vi "Compute DistanceToTarget2.vi"(8 "Rect":T1, 9 "Camera Type":T3, 11 "Image Src":T2) -> (2 "Distance (ft)":dbl, 3 "Image Dst Out":T2)   [LabVIEW 2025]
doc: "Using the camera lens information and the real world size of the target, use trig and ratios to determine the distance to the target. Also returns the location relative to the image center in a (-1 , 1) coordinate system that may be useful for steering the robot."
uses:
  Camera Types.ctl
  <vilib>/vision/Image Controls.llb/IMAQ Image.ctl
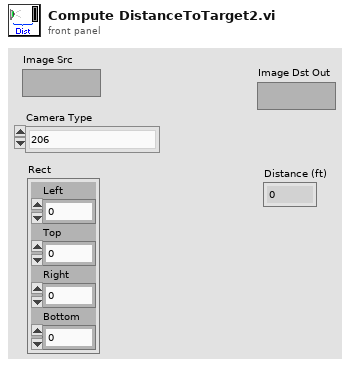
[diagram p1: front panel]
types:
  T1 = cluster{"Left":dbl, "Top":dbl, "Right":dbl, "Bottom":dbl}
  T2 = typedef "IMAQ Image.ctl" = refnum<image>
  T3 = typedef "Camera Types.ctl" = enum16{"206", "1011", "1013", "MS HD3000 square", "MS HD3000 640x480"}
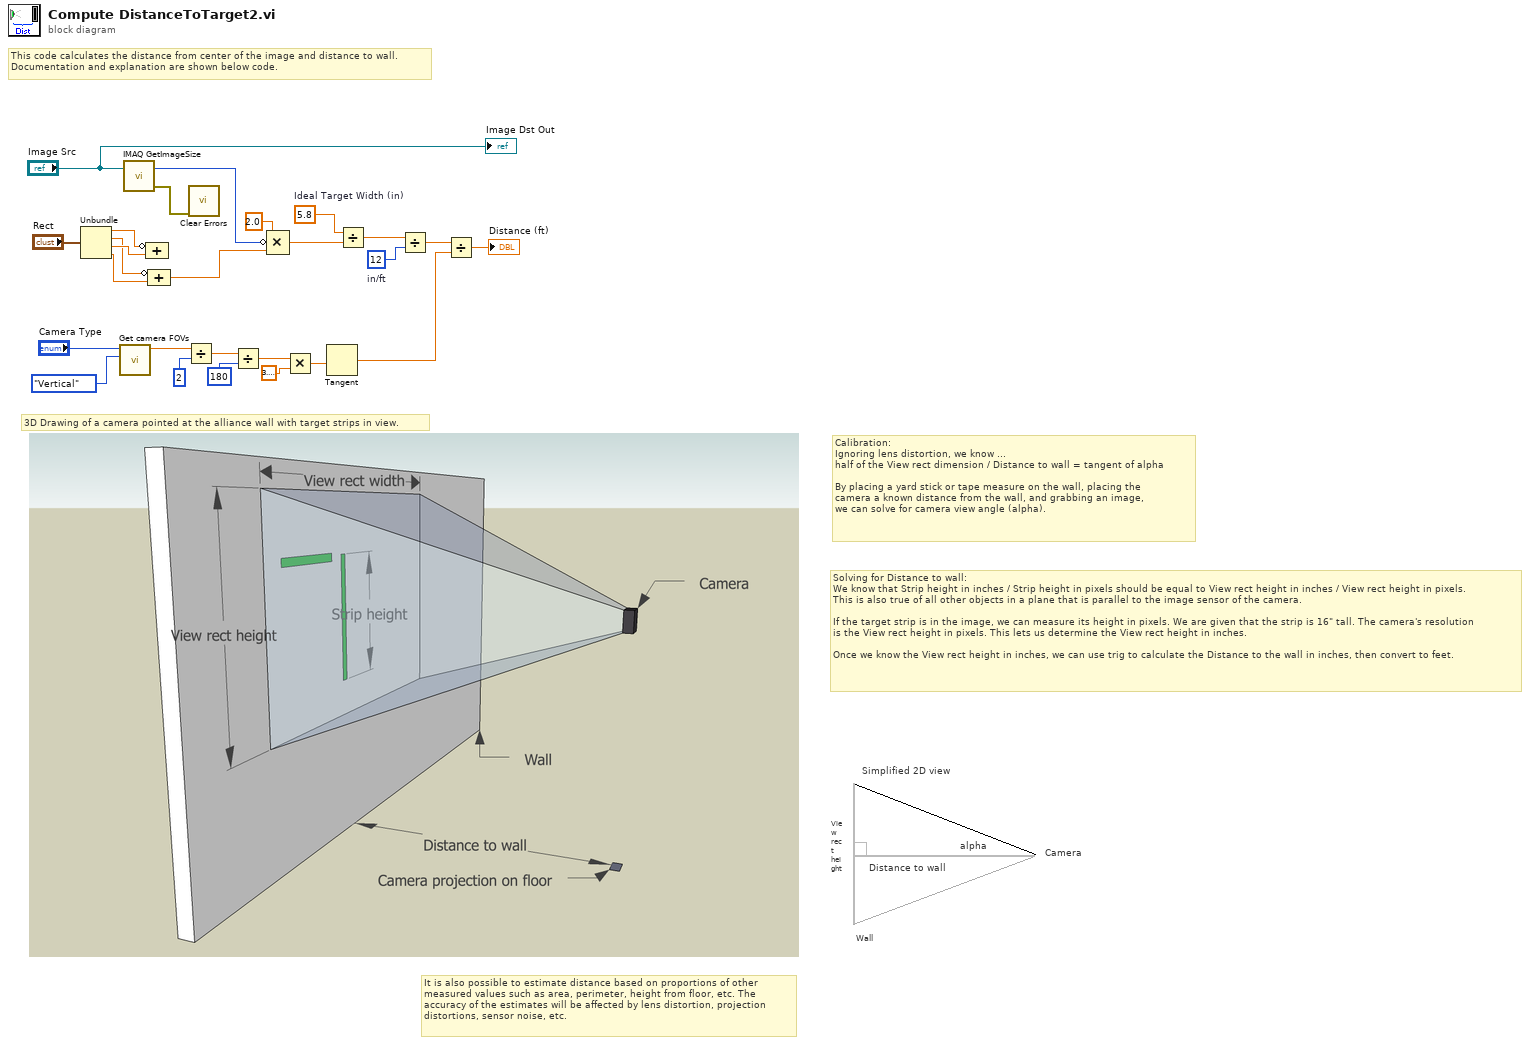
[diagram p0: block diagram]
diagram:
  w15 = 5.8  # Ideal Target Width (in)
  w20 = 12  # in/ft
  # "It is also possible to estimate distance based on proportions of other\nmeasured values such as area, perimeter, height from floor, etc. The\naccuracy of the estimates will be affected by lens distortion, projection\ndistortions, sensor noise, etc."
  # "Wall"
  # "Camera"
  # "Simplified 2D view"
  # "Solving for Distance to wall:\nWe know that Strip height in inches / Strip height in pixels should be equal to View rect height in inches / View rect height in pixels.\nThis is also true of all other objects in a plane that is parallel to the image sensor of the camera.\n\nIf the target strip is in the image, we can measure its height in pixels. We are given that the strip is 16\" tall. The camera's resolution\nis the View rect height in pixels. This lets us determine the View rect height in inches.\n\nOnce we know the View rect height in inches, we can use trig to calculate the Distance to the wall in inches, then convert to feet."
  # "3D Drawing of a camera pointed at the alliance wall with target strips in view."
  # "Distance to wall"
  # "View rect height"
  # "alpha"
  # "Calibration:\nIgnoring lens distortion, we know ...\nhalf of the View rect dimension / Distance to wall = tangent of alpha\n\nBy placing a yard stick or tape measure on the wall, placing the\ncamera a known distance from the wall, and grabbing an image,\nwe can solve for camera view angle (alpha)."
  # "This code calculates the distance from center of the image and distance to wall.\nDocumentation and explanation are shown below code."
  n1 = Unbundle("Rect") -> ("Left"=w5:dbl, "Top"=w3:dbl, "Right"=w4:dbl, "Bottom"=w2:dbl)
  n2 = call "Get camera FOVs.vi"("Type"=enum16{"Horizontal", "Vertical", "Diagonal"}."Vertical" ("Angle"), "Camera Type"="Camera Type") -> ("FOV"=w17:dbl)  [unwired: 8 in, 1 out]
  n3 = call "IMAQ GetImageSize"("Image"="Image Src") -> ("Y Resolution"=w12:i32, "error out"=w11:errorcluster)  [unwired: 3 in, 1 out]
  n4 = Compound Arithmetic op=ADD(invert w5, w4) -> ()  [unwired: 1 out]
  n5 = Compound Arithmetic op=ADD(invert w3, w2) -> (w1:dbl)
  n6 = Divide(x=w17, y=2) -> (x/y=w23:dbl)
  n7 = call <vilib>:"Clear Errors.vi"("error in (no error)"=w11) -> ()  [unwired: 5 in, 2 out]
  n8 = Divide(x=w23, y=180) -> (x/y=w22:dbl)
  n9 = Compound Arithmetic op=MULTIPLY(2.0, invert w12, w1) -> (w13:dbl)
  n10 = Multiply(x=w22, y=3.141592653589793) -> (x*y=w24:dbl)
  n11 = Tangent(1:w24) -> (0:w19:dbl)
  n12 = Divide(x=w15, y=w13) -> (x/y=w6:dbl)
  n13 = Divide(x=w6, y=w20) -> (x/y=w18:dbl)
  n14 = Divide(x=w18, y=w19) -> (x/y=→"Distance (ft)":dbl)
  "Image Dst Out" <- "Image Src"
